vi "CSM - Configuration File Path.vi"(5 "Include All Paths? (F)":bool, 8 "error in (no error)":errorcluster) -> (1 "All Config Files":path[](array[path]), 2 "error out":errorcluster, 3 "Default Config File Path":path)   [LabVIEW 2017, in "INI-Static-Variable-Support.lvlib"]
doc: "Returns the paths of all loaded configuration files.\n\n<b>Reference Example</b>: `5. import Config.ini with __include section.vi`.\n\n\n> [!NOTE] <b>CSM INI-Variable Configuration File Path</b>\n>\n> - <b>Development State</b>: The first INI configuration file found in the Application Directory. If no configuration file exists, it defaults to `csm-app.ini`.\n> - <b>Post-Compilation</b>: An INI configuration file in the same directory as the executable file, with the same name as the executable. LabVIEW automatically generates this file after compilation.\n> - Supports loading multiple configuration files. Configuration items in files loaded later will overwrite identical items in previously loaded files.\n> - Configuration files can use the `[__include]` section to reference other configuration files.\n> - Supports both relative and absolute paths.\n> - Relative paths are relative to the path of the current configuration file.\n> - The name of the configuration file in the `[__include]` section is not critical, as long as the path is correct.\n> - To avoid circular references, the same configuration file will be automatically ignored if loaded a second time.\n\n\n-- <b>Controls</b> --\n- <b>Include All Paths?(F)</b>: Whether to include all configuration file paths.\n\n-- <b>Indicators</b> --\n- <b>Default Config File Path</b>: Default configuration file path.\n- <b>All Config Files</b>: List of all configuration files."
uses:
  INI-Static-Variable-Support.lvlib
  _Support/_fgv-oper.ctl
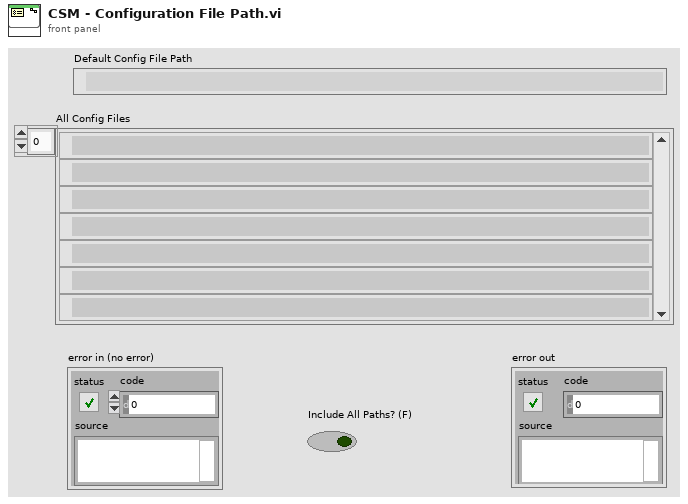
[diagram p1: front panel]
types:
  T1 = typedef "INI-Static-Variable-Support.lvlib/_fgv-oper.ctl" = enum16{"Read", "Write", "Sync", "Sessions", "List Keys", "Load", "List Files", "List Variables", "List Permanent Variables", "Mark Temp Variable as Permenent", "unload", "INIConfig(Memory)", "Reset", "Restore Variable Value", "Load From String"}
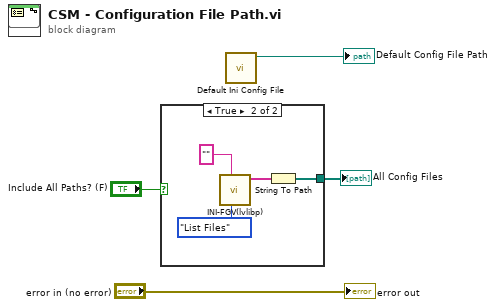
[diagram p0: block diagram]
diagram:
  n1 = case shown="True" "Include All Paths? (F)" {
    tunnel: [_ w6] -> w2
    frame False {
    }
    frame True {
      n2 = call "INI-FGV(lvlibp).vi"("Enum"=_fgv-oper."List Files", "Prefered Section"="") -> ("Array"=w7:string[])  [unwired: 6 in, 3 out]
      n3 = String To Path(string=w7) -> (path=w6:path[])
    }
  }
  "All Config Files" <- w2
  n4 = call "Default Ini Config File.vi"() -> ("appended path"=→"Default Config File Path":path)  [unwired: 11 in]
  "error out" <- "error in (no error)"
